vi "sinus.vi"(11 "x [rad]":dbl) -> (3 "sin(x)":dbl)   [LabVIEW 2017]
uses:
  <vilib>/gmath/NI_Gmath.lvlib
panel:
  out "sin(x) lib":dbl
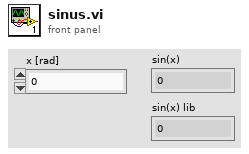
[diagram p1: front panel]
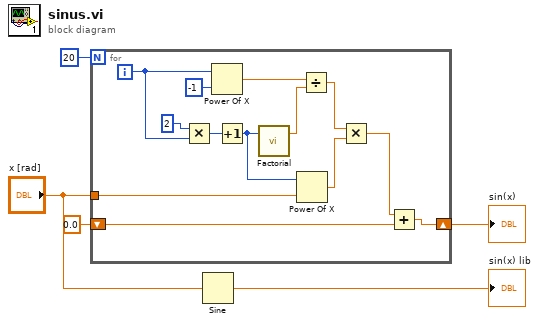
[diagram p0: block diagram]
diagram:
  n1 = for {
    N: 20 -> [_]
    shift-right: [w7] -> w3
    shift-left: 0.0 -> [w8]
    tunnel: "x [rad]" -> [w6]
    i -> [w14]
    n2 = Multiply(x=2, y=w14) -> (x*y=w15:i32)
    n3 = Power Of X(1:-1 ("x"), 2:w14) -> (0:w17:dbl)
    n4 = Increment(x=w15) -> (x+1=w10:i32)
    n5 = call <vilib>:"Factorial.vi"("n"=w10) -> ("n!"=w13:dbl)  [unwired: 2 in]
    n6 = Power Of X(1:w6, 2:w10) -> (0:w11:dbl)
    n7 = Divide(x=w17, y=w13) -> (x/y=w12:dbl)
    n8 = Multiply(x=w12, y=w11) -> (x*y=w9:dbl)
    n9 = Add(x=w9, y=w8) -> (x+y=w7:dbl)
  }
  "sin(x)" <- w3
  n10 = Sine(x="x [rad]") -> (sin(x)=→"sin(x) lib":dbl)
